vi "Serialize - JSON.vi"(8 "error in":errorcluster, 11 "SOAP Data in":refnum<class "SOAP Data.lvclass">) -> (0 "error out":errorcluster, 2 "Serialized JSON":string, 3 "SOAP Data out":refnum<class "SOAP Data.lvclass">)   [LabVIEW 2017, in "Controller.lvlib" / "SOAP Data.lvclass"]
uses:
  SOAP Data.lvclass
  SOAP Data.lvclass/SOAP Data.ctl
  <vilib>/MSR Consulting, LLC/General Reuse/Data/Data.lvclass
  Heater Data/Heater Data.lvclass
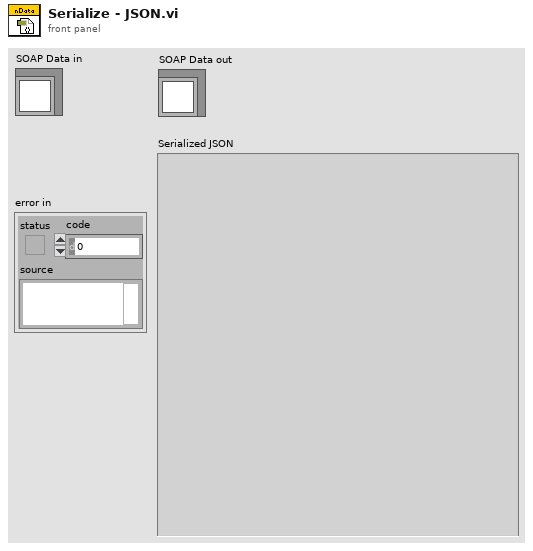
[diagram p1: front panel]
types:
  T1 = cluster{"pas_cell_1":sgl, "pas_cell_2":sgl, "pas_las_head_1":sgl, "pas_las_head_2":sgl, "box_exit":sgl, "crd_heater":sgl, "box_inlet":sgl, "crd_laser_head":sgl, "cjc":sgl, "autozero":sgl}
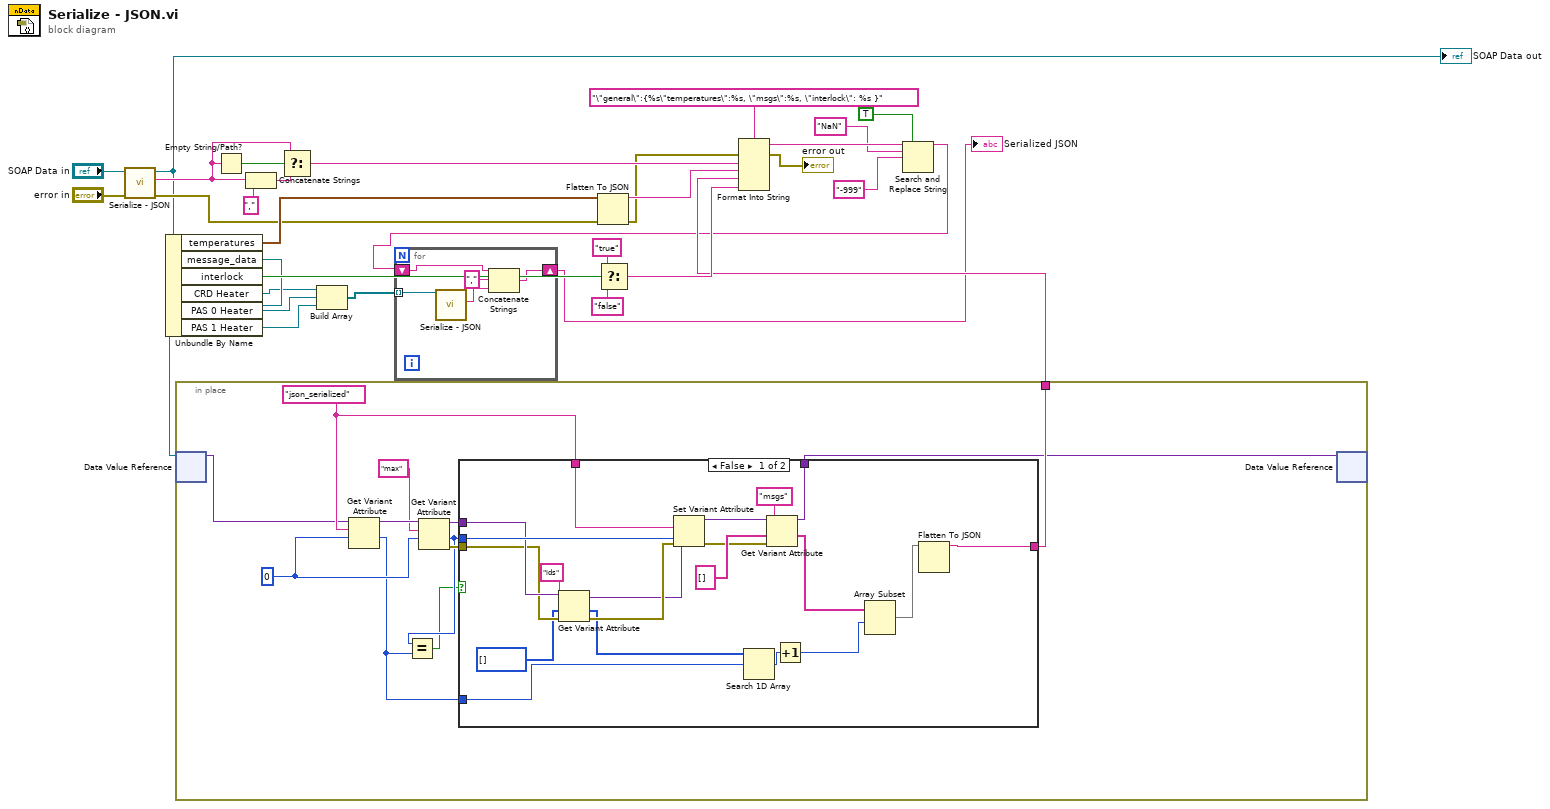
[diagram p0: block diagram]
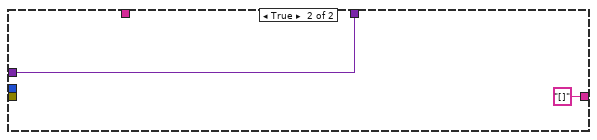
[diagram p2: hidden frame]
diagram:
  n1 = call-parent "Serialize - JSON.vi"("error in"="error in", "Data in"="SOAP Data in") -> ("error out"=w20:errorcluster, "Serialized JSON"=w26:string, "Data out"=w12:refnum<class "SOAP Data.lvclass">)  [unwired: 7 in]
  "SOAP Data out" <- w12
  n2 = Unbundle By Name(w12) -> ("temperatures"=w21:T1, "message_data"=w11:refnum<data-value>, "interlock"=w15:bool, "CRD Heater"=w6:refnum<class "Heater Data.lvclass">, "PAS 0 Heater"=w5:refnum<class "Heater Data.lvclass">, "PAS 1 Heater"=w4:refnum<class "Heater Data.lvclass">)
  n3 = in-place {
    in-place-border: [w34] -> w14
    w40 = u64 0
    w39 = "json_serialized" ("name")
    n4 = in-place-dvr #1(w11) -> (w32:variant)  [unwired: 1 out]
    n5 = Get Variant Attribute(Variant=w32, name=w39, default value (empty Variant)=w40) -> (duplicate Variant=w42:variant, value=w33:u64)  [unwired: 1 in, 2 out]
    n6 = Get Variant Attribute(Variant=w42, name="max", default value (empty Variant)=w40) -> (duplicate Variant=w38:variant, value=w36:u64, error out=w37:errorcluster)  [unwired: 1 in, 1 out]
    n7 = Equal?(x=w36, y=w33) -> (x = y?=w35:bool)
    n8 = case shown="False" w35 {
      tunnel: w39 -> [w62 _]
      tunnel: w36 -> [w61 _]
      tunnel: w38 -> [w60 w63]
      tunnel: w37 -> [w59 _]
      tunnel: [w51 "[]" ("JSON string")] -> w34
      tunnel: w33 -> [w48 _]
      tunnel: [w43 w63] -> w31
      frame False {
        n9 = Get Variant Attribute(Variant=w60, name="ids", default value (empty Variant)=u64[] [], error in=w59) -> (duplicate Variant=w56:variant, value=w49:u64[], error out=w57:errorcluster)  [unwired: 1 out]
        n10 = Set Variant Attribute(Variant=w56, name=w62, value=w61, error in=w57) -> (Variant out=w52:variant, error out=w50:errorcluster)  [unwired: 1 out]
        n11 = Search 1D Array(1D array=w49, element=w48) -> (index of element=w46:i32)  [unwired: 1 in]
        n12 = Get Variant Attribute(Variant=w52, name="msgs", default value (empty Variant)=string[] [], error in=w50) -> (duplicate Variant=w43:variant, value=w47:string[])  [unwired: 2 out]
        n13 = Increment(x=w46) -> (x+1=w45:i32)
        n14 = Array Subset(array=w47, index=w45) -> (w44:string[])  [unwired: 1 in]
        n15 = Flatten To JSON(anything=w44) -> (JSON string=w51:string)  [unwired: 2 in, 1 out]
      }
      frame True {
      }
    }
    n16 = in-place-dvr #1(w31) -> ()  [unwired: 2 out]
  }
  n17 = Empty String/Path?(string/path=w26) -> (empty?=w28:bool)
  n18 = Concatenate Strings(w26, "," ("string")) -> (w27:string)
  n19 = Select(t=w26, s=w28, f=w27) -> (s? t:f=w23:string)
  n20 = Build Array(w6, w5, w4) -> (w3:refnum<class "Heater Data.lvclass">[])
  n21 = Flatten To JSON(anything=w21, error in (no error)=w20) -> (JSON string=w22:string, 11:w13:errorcluster)  [unwired: 1 in]
  n22 = Select(t="true", s=w15, f="false") -> (s? t:f=w16:string)
  n23 = Format Into String(format string="\"general\":{%s\"temperatures\":%s, \"msgs\":%s, \"interlock\": %s }", error in=w13, w23, w22, w14, w16) -> (resulting string=w9:string, error out=→"error out":errorcluster)  [unwired: 1 in]
  n24 = Search and Replace String(replace all?=TRUE ("replace all? (F)"), input string=w9, search string="NaN", replace string="-999" ("replace string (\"\")")) -> (result string=w2:string)  [unwired: 4 in, 3 out]
  n25 = for {
    tunnel: w3 -> [w69] mode=indexing
    shift-right: [w65] -> w1
    shift-left: w2 -> [w66]
    n26 = call-dynamic "Serialize - JSON.vi"("Heater Data in"=w69) -> ("Serialized JSON"=w68:string)  [unwired: 8 in, 2 out]
    n27 = Concatenate Strings(w66, "," ("string"), w68) -> (w65:string)
  }
  "Serialized JSON" <- w1
